vi "Connect Matching Terminal Names.vi"(8 "error in (no error)":errorcluster, 10 "Terminal Set #2":refnum<vi>[](array[refnum]), 11 "Terminal Set #1":refnum<vi>[](array[refnum])) -> (0 "error out":errorcluster)   [LabVIEW 2016, in "SLL Scripting.lvlib" / "SLL Class DVR API Generator.lvlib"]
uses:
  SLL Class DVR API Generator.lvlib
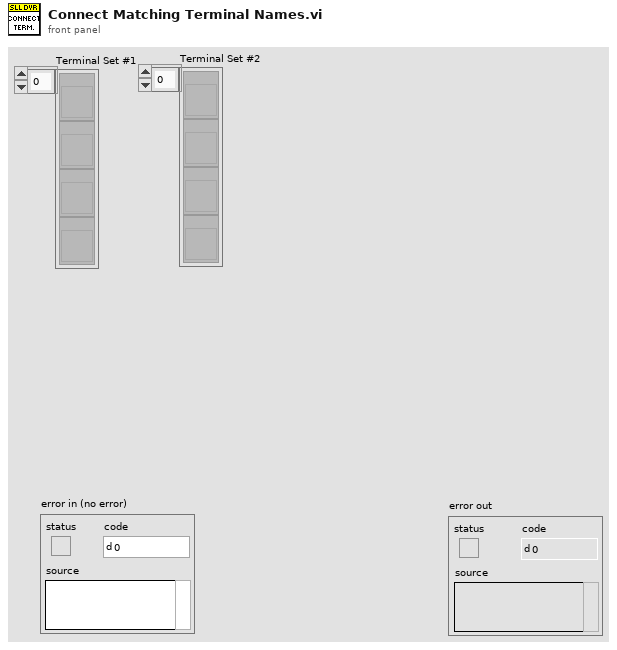
[diagram p1: front panel]
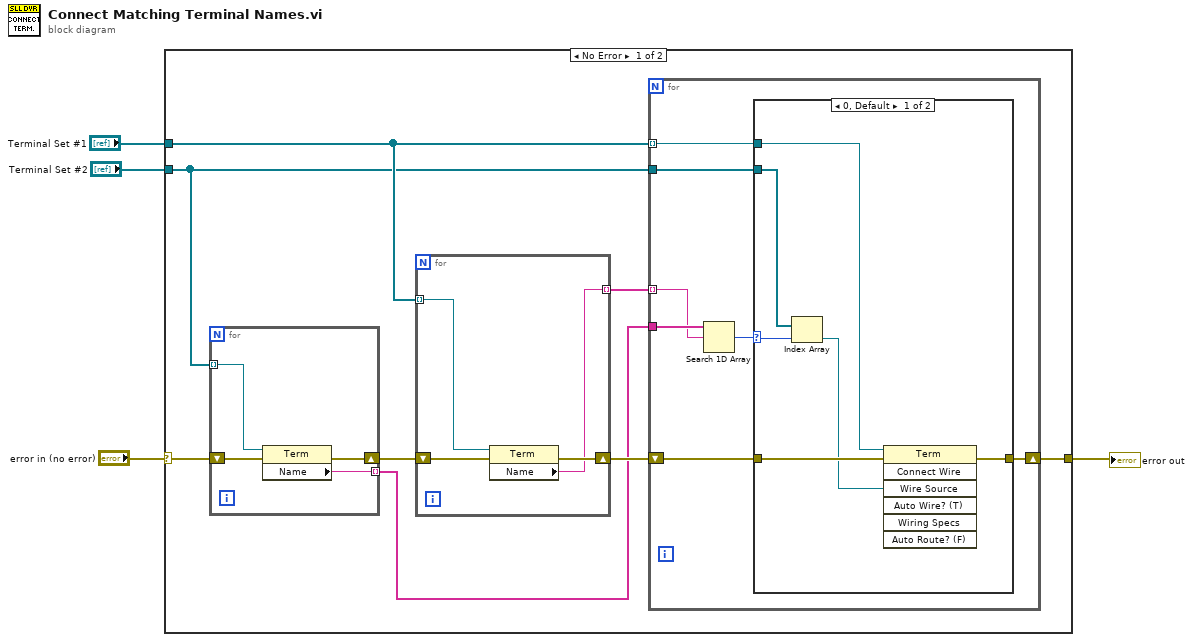
[diagram p0: block diagram]
diagram:
  n1 = case shown="No Error" "error in (no error)" {
    selector: "error in (no error)" -> [w12 w35]
    tunnel: [w9 w35] -> w3
    tunnel: "Terminal Set #1" -> [w6 _]
    tunnel: "Terminal Set #2" -> [w5 _]
    frame No Error {
      n2 = for {
        shift-right: [w29] -> w10
        shift-left: w12 -> [w30]
        tunnel: w5 -> [w28] mode=indexing
        tunnel: [w27] -> w7 mode=indexing
        n3 = property class="Term"(reference=w28, error in=w30) -> (error out=w29:errorcluster, "Name"=w27:string)  [unwired: 1 out]
      }
      n4 = for {
        shift-right: [w33] -> w11
        shift-left: w10 -> [w34]
        tunnel: w6 -> [w32] mode=indexing
        tunnel: [w31] -> w8 mode=indexing
        n5 = property class="Term"(reference=w32, error in=w34) -> (error out=w33:errorcluster, "Name"=w31:string)  [unwired: 1 out]
      }
      n6 = for {
        shift-right: [w18] -> w9
        shift-left: w11 -> [w19]
        tunnel: w8 -> [w16] mode=indexing
        tunnel: w7 -> [w17]
        tunnel: w6 -> [w14] mode=indexing
        tunnel: w5 -> [w13]
        n7 = Search 1D Array(1D array=w17, element=w16) -> (index of element=w15:i32)  [unwired: 1 in]
        n8 = case shown="0, Default" w15 {
          selector: w15 -> [w21 _]
          tunnel: w19 -> [w25 w26]
          tunnel: [w24 w26] -> w18
          tunnel: w14 -> [w23 _]
          tunnel: w13 -> [w22 _]
          frame 0, Default {
            n9 = Index Array(array=w22, index=w21) -> (element=w20:refnum<vi>)
            n10 = invoke class="Term" method="Connect Wire"(reference=w23, error in=w25, "Wire Source"=w20) -> (error out=w24:errorcluster)  [unwired: 4 in, 6 out]
          }
          frame -1 {
          }
        }
      }
    }
    frame Error {
    }
  }
  "error out" <- w3
